vi "Write RT FIFO(16B).vi"(6 "overwrite on timeout (T)":bool, 7 "FIFO Options":T1, 8 "error in (no error)":errorcluster, 9 "timeout in ms (0)":i32, 10 "element":T3, 11 "RT FIFO in":T2) -> (0 "error out":errorcluster, 1 "timed out?":bool, 3 "RT FIFO out":T2)   [LabVIEW 2017, in "DSF Core.lvlib" / "Interface.lvclass"]
uses:
  Interface.lvclass
  RT FIFO Data 16B.ctl
  RT FIFO Payload 16B.ctl
  RT FIFO Ref 16B.ctl
  Typedefs/FIFO Flags.ctl
  DSF Core.lvlib
panel:
  out "# elements":u32
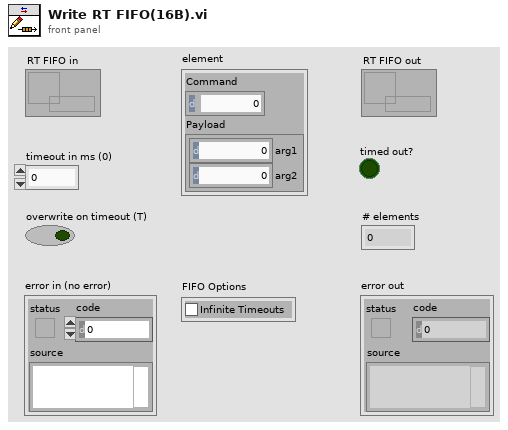
[diagram p1: front panel]
types:
  T1 = typedef "DSF Core.lvlib/FIFO Flags.ctl" = cluster{"Infinite Timeouts":bool}
  T2 = typedef "DSF Core.lvlib/Interface.lvclass/RT FIFO Ref 16B.ctl" = refnum<k33>
  T3 = typedef "DSF Core.lvlib/Interface.lvclass/RT FIFO Data 16B.ctl" = cluster{"Command":u8, "Payload":T4}
  T4 = typedef "DSF Core.lvlib/Interface.lvclass/RT FIFO Payload 16B.ctl" = cluster{"arg1":u64, "arg2":u64}
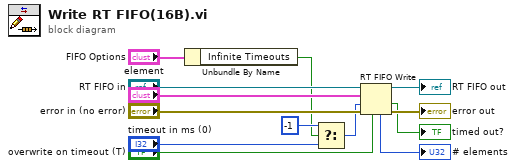
[diagram p0: block diagram]
diagram:
  n1 = Unbundle By Name("FIFO Options") -> ("Infinite Timeouts"=w1:bool)
  n2 = Select(t=-1, s=w1, f="timeout in ms (0)") -> (s? t:f=w4:i32)
  n3 = RT FIFO Write(0:"RT FIFO in", 1:"element", 2:w4, 3:"error in (no error)", 5:"overwrite on timeout (T)") -> (7:→"# elements":u32, 8:→"RT FIFO out":T2, 10:→"timed out?":bool, 11:→"error out":errorcluster)
